vi "Move Objects Demo - Handle Object Movements.vi"(8 "error in (no error)":errorcluster) -> (0 "error out":errorcluster)   [LabVIEW 2012]
doc: "This is a background process that will communicate with UI and handle the object movements. It will communicate with OBJECT Queue."
uses:
  Controls/Global Stop States.ctl
  <vilib>/Utility/inputDevices.llb/closeMouse.vi
  <vilib>/Utility/inputDevices.llb/mouseAcquire.vi
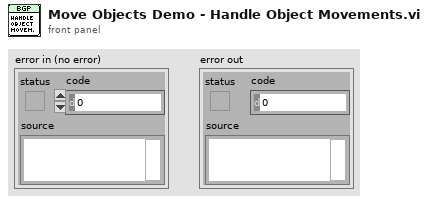
[diagram p1: front panel]
types:
  T1 = typedef "Global Stop States.ctl" = enum16{"STOP", "STATUS", "INIT"}
  T2 = typedef "LVPositionTypeDef.ctl" = cluster{"Left":i32, "Top":i32}
  T3 = cluster{"Horizontal":i32, "Vertical":i32, "Scrolling":i32}
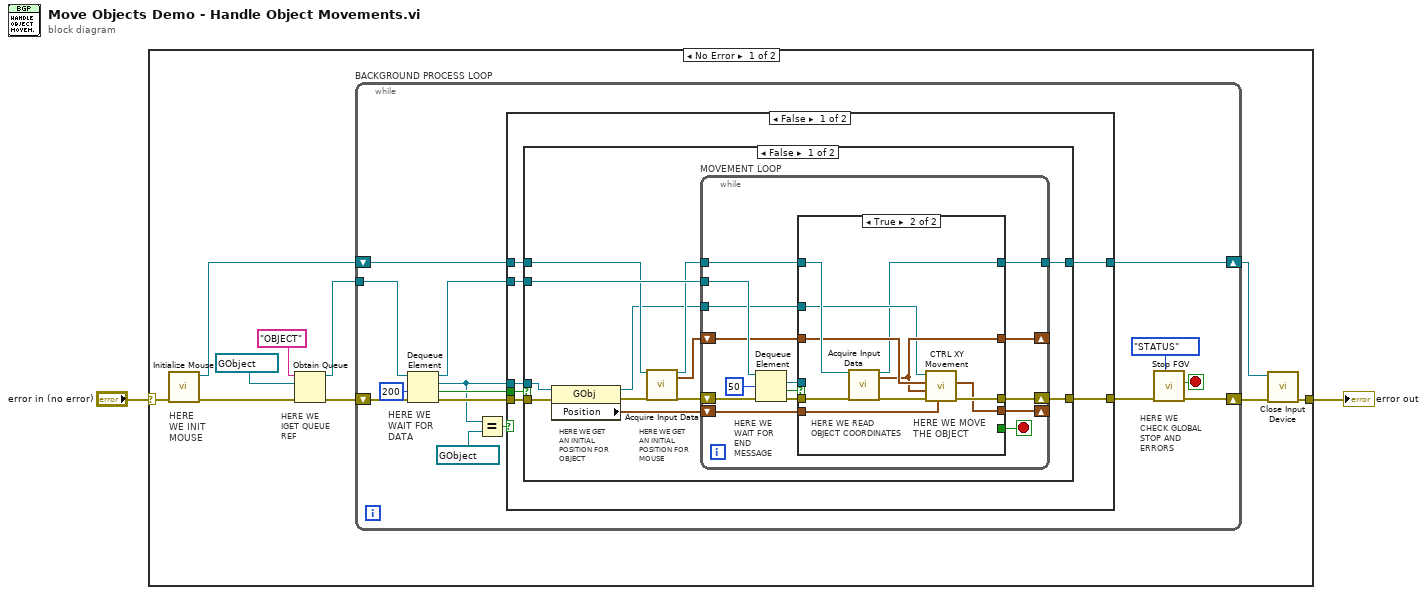
[diagram p0: block diagram]
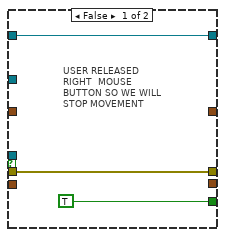
[diagram p2: hidden frame]
diagram:
  n1 = case shown="No Error" "error in (no error)" {
    selector: "error in (no error)" -> [w3 w79]
    tunnel: [w7 w79] -> w2
    frame No Error {
      # "HERE WE IGET QUEUE REF"
      # "HERE WE INIT MOUSE"
      n2 = call <vilib>:"Initialize Mouse.vi"("error in (no error)"=w3) -> ("error out"=w4:errorcluster, "device ID"=w12:refnum<k1>)  [unwired: 9 in]
      n3 = Obtain Queue(name (unnamed)="OBJECT", element data type=refnum<vi> refnum ("reference out"), error in (no error)=w4) -> (queue out=w9:refnum<queue>, error out=w5:errorcluster)  [unwired: 2 in, 1 out]
      n4 = while "BACKGROUND PROCESS LOOP" {
        tunnel: w9 -> [w27]
        shift-right: [w19] -> w8
        shift-left: w5 -> [w26]
        shift-right: [w20] -> w6
        shift-left: w12 -> [w21]
        stop <- w17 stop-if-true
        # "HERE WE WAIT FOR  DATA"
        # "HERE WE CHECK GLOBAL STOP AND ERRORS"
        n5 = Dequeue Element(queue=w27, timeout in ms (-1)=200, error in (no error)=w26) -> (queue out=w22:refnum<queue>, element=w14:refnum<vi>, timed out?=w23:bool, error out=w25:errorcluster)
        n6 = Equal?(x=w14, y=refnum<vi> refnum ("reference out")) -> (x = y?=w13:bool)
        n7 = case shown="False" w13 {
          tunnel: w25 -> [w34 w78]
          tunnel: w23 -> [w33 _]
          tunnel: w22 -> [w32 _]
          tunnel: w21 -> [w31 w77]
          tunnel: [w30 w77] -> w20
          tunnel: [w29 w78] -> w18
          tunnel: w14 -> [w28 _]
          frame False {
            n8 = case shown="False" w33 {
              tunnel: w28 -> [w37 _]
              tunnel: w34 -> [w36 w76]
              tunnel: [w44 w76] -> w29
              tunnel: w32 -> [w45 _]
              tunnel: w31 -> [w40 w75]
              tunnel: [w35 w75] -> w30
              frame False {
                # "HERE WE GET AN INITIAL POSITION FOR MOUSE"
                # "HERE WE GET AN INITIAL POSITION FOR OBJECT"
                n9 = property class="GObj"(reference=w37, error in=w36) -> (reference out=w38:refnum<vi>, error out=w43:errorcluster, "Position"=w46:T2)
                n10 = call-poly <vilib>:"Acquire Input Data.vi"("device ID"=w40, "error in (no error)"=w43) -> ("device ID"=w39:refnum<k1>, "axis info"=w41:T3, "error out"=w42:errorcluster)  [unwired: 14 in, 1 out]
                n11 = while "MOVEMENT LOOP" {
                  shift-right: [w53] -> w44
                  shift-left: w42 -> [w61]
                  tunnel: w45 -> [w60]
                  tunnel: w39 -> [w54]
                  shift-right: [w49] -> _
                  shift-left: w41 -> [w51]
                  shift-right: [w50] -> _
                  shift-left: w46 -> [w52]
                  tunnel: w38 -> [w48]
                  tunnel: [w47] -> w35
                  stop <- w56 stop-if-true
                  # "HERE WE WAIT FOR END MESSAGE"
                  n12 = Dequeue Element(queue=w60, timeout in ms (-1)=50, error in (no error)=w61) -> (element=w55:refnum<vi>, timed out?=w58:bool, error out=w57:errorcluster)  [unwired: 1 out]
                  n13 = case shown="True" w58 {
                    tunnel: w57 -> [w63 w74]
                    tunnel: [TRUE _] -> w56
                    tunnel: w55 -> [_ _]
                    tunnel: w54 -> [w62 w73]
                    tunnel: [w63 w69] -> w53
                    tunnel: w52 -> [_ w68]
                    tunnel: w51 -> [_ w72]
                    tunnel: [_ w67] -> w50
                    tunnel: [_ w71] -> w49
                    tunnel: w48 -> [_ w66]
                    tunnel: [w62 w65] -> w47
                    frame False {
                      # "USER RELEASED RIGHT  MOUSE BUTTON SO WE WILL STOP MOVEMENT"
                    }
                    frame True {
                      # "HERE WE MOVE THE OBJECT"
                      # "HERE WE READ OBJECT COORDINATES"
                      n14 = call-poly <vilib>:"Acquire Input Data.vi"("device ID"=w73, "error in (no error)"=w74) -> ("device ID"=w65:refnum<k1>, "axis info"=w71:T3, "error out"=w70:errorcluster)  [unwired: 14 in, 1 out]
                      n15 = call "CTRL XY Movement.vi"("Position in"=w68, "error in"=w70, "Current Axis Info In"=w71, "Previous Axis Info In"=w72, "Ref In"=w66) -> ("error out"=w69:errorcluster, "Position out"=w67:T2)  [unwired: 5 in]
                    }
                  }
                }
              }
              frame True {
                # "TIMED OUT"
              }
            }
          }
          frame True {
            # "NOT A GOBJECT SO WE DON'T DO ANYTHING HERE"
          }
        }
        n16 = call "Stop FGV.vi"("Operation In"=Global_Stop_States."STATUS", "error in"=w18) -> ("error out"=w19:errorcluster, "Stop?"=w17:bool)  [unwired: 8 in]
      }
      n17 = call-poly <vilib>:"Close Input Device.vi"("error in (no error)"=w8, "device ID"=w6) -> ("error out"=w7:errorcluster)  [unwired: 8 in]
    }
    frame Error {
    }
  }
  "error out" <- w2
